vi "Convert I2C Messages.vi"(8 "error in (no error)":errorcluster, 11 "I2C Messages":string[][](array[string])) -> (0 "error out":errorcluster, 3 "U64 Array":u64[](array[numeric]))   [LabVIEW 2025, in "I2C Bus Monitor.lvclass"]
uses:
  I2C Bus Monitor.lvclass
  I2C Bus Monitor.lvclass/I2C Bus Monitor.ctl
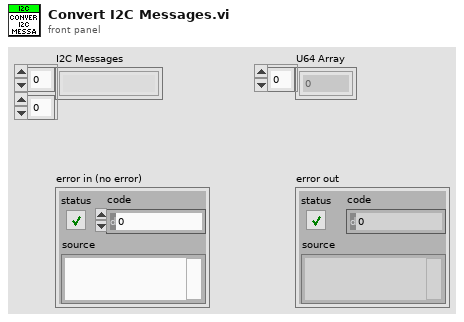
[diagram p1: front panel]
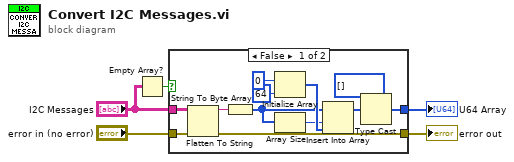
[diagram p0: block diagram]
diagram:
  n1 = Empty Array?(array="I2C Messages") -> (empty?=w2:bool)
  n2 = case shown="False" w2 {
    tunnel: "error in (no error)" -> [w17 w18]
    tunnel: [w16 w18] -> w4
    tunnel: [w15 _] -> w3
    tunnel: "I2C Messages" -> [w13 _]
    frame False {
      n3 = Flatten To String(anything=w13, error in (no error)=w17) -> (data string=w12:string, error out=w16:errorcluster)  [unwired: 2 in, 1 out]
      n4 = String To Byte Array(string=w12) -> (unsigned byte array=w7:u8[])
      n5 = Initialize Array(u8 0, 64 ("y")) -> (w10:u8[])
      n6 = Array Size(array=w7) -> (size(s)=w6:i32)
      n7 = Insert Into Array(array=w7, index=w6, new element=w10) -> (w11:u8[])
      n8 = Type Cast(type=u64[] [], x=w11) -> (*(type *) &x=w15:u64[])
    }
    frame True {
    }
  }
  "error out" <- w4
  "U64 Array" <- w3
